vi "INTERFACE.EDIBON.vi"() -> ()   [LabVIEW 2014]
uses:
  Global 5.vi
  <vilib>/measure/madcrms.llb/Basic Averaged DC-RMS for N Chan.vi
  Global 2.vi
  <vilib>/measure/NI_MAPro.lvlib
  <vilib>/Analysis/NI_AALPro.lvlib
panel:
  out "?":dbl format="%#_3f"
  out "?":dbl format="%#_3f"
  out "SRL-1":dbl format="%#_5f"
  out "ST-3":dbl format="%#_4f"
  out "ST-2":dbl format="%#_4f"
  out "V_DC":dbl format="%#_3f"
  out "I_DC":dbl format="%#_3f"
  out "ST-1":dbl format="%#_4f"
  out "I_DC":dbl format="%#_3f"
  out "V_DC":dbl format="%#_3f"
  in  "SOL 2":dbl(slide) min=0.0 max=10.0 step=2.0 scale=0.0..10.0 scale format="%#_1f"
  in  "chave sol2":bool
  in  "chave sol1":bool
  in  "MEAS":bool
  in  "VENTILADORES":bool
  in  "SÉRIE-PARALELO":bool
  out "SRL-1":dbl format="%#_5f"
  out "ST-3":dbl format="%#_4f"
  out "ST-2":dbl format="%#_4f"
  out "ST-1":dbl format="%#_4f"
  in  "PAINEL 2":bool
  in  "PAINEL 1":bool
  in  "SOL 1":dbl(slide) min=0.0 max=10.0 step=2.0 scale=0.0..10.0 scale format="%#_1f"
  in  "stop":bool
  out "Tempo de salvamento (sec)":dbl format="%.1f"
  in  "OK Button":bool
  in  "COMEÇAR":bool
  in  "quit? (T)":bool
  in  "?":bool
  in  "PLOTE NO GRÁFICO:":u16(ring) items=["GRÁFICO A", "GRÁFICO B", "GRÁFICO ÚNICO"]
  in  "I_DC":bool
  in  "ST_2":bool
  in  "ST_1":bool
  in  "V_DC":bool
  in  "ST_3":bool
  in  "SRL_1":bool
  in  "I_DC":bool
  in  "ST_2":bool
  in  "ST_1":bool
  in  "V_DC":bool
  in  "ST_3":bool
  in  "SRL_1":bool
  out "GRÁFICO B":cluster{dbl[], dbl[]}[](graph)
  out "GRÁFICO A":cluster{dbl[], dbl[]}[](graph)
  out "GRÁFICO ÚNICO":cluster{dbl[], dbl[]}[](graph)
  in  "I_DC":bool
  in  "ST_2":bool
  in  "ST_1":bool
  in  "V_DC":bool
  in  "ST_3":bool
  in  "SRL_1":bool
  # "POTENCIA DE SAIDA"
  # "W"
  # "ºC"
  # "ºC"
  # "ºC"
  # "W/m2"
  # "V"
  # "A"
  # "PLOTE O SENSOR:"
  # "ANTES"
  # "DEPOIS"
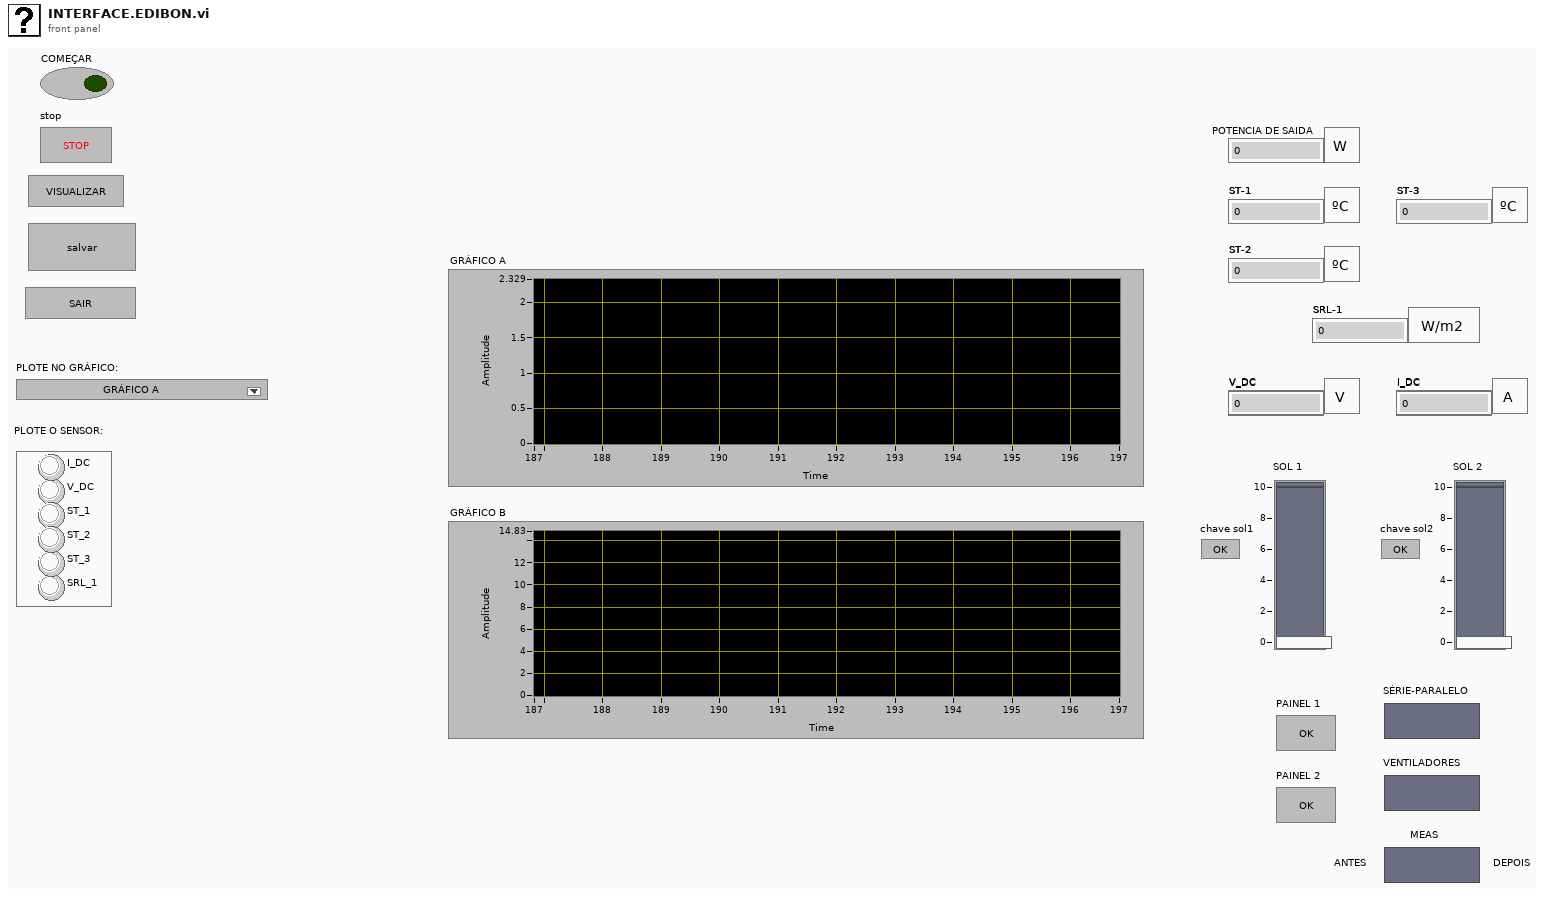
[diagram p1: front panel]
types:
  T1 = enum32{"Invalid", "Standard", "Closed", "Hidden", "Minimized", "Maximized"}
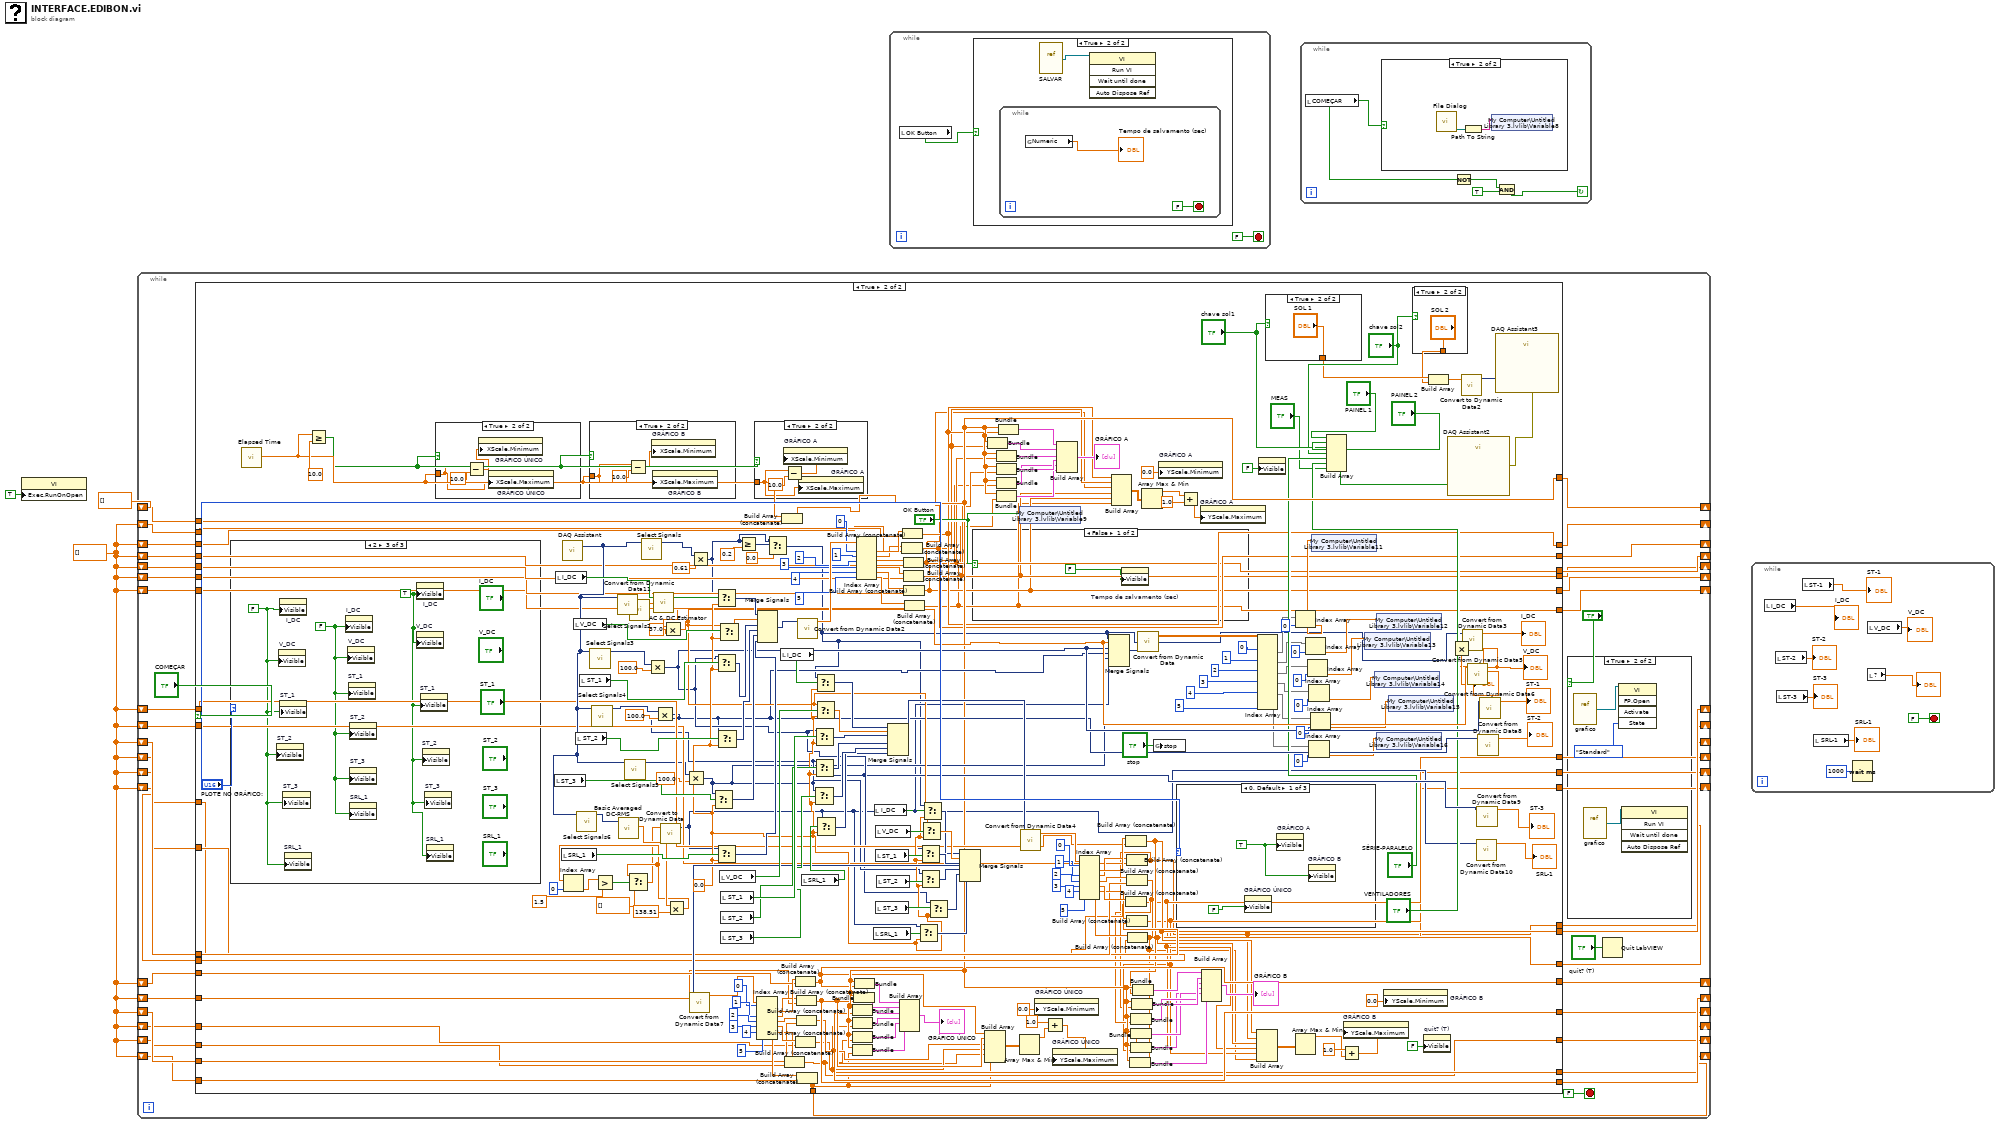
[diagram p0: block diagram]
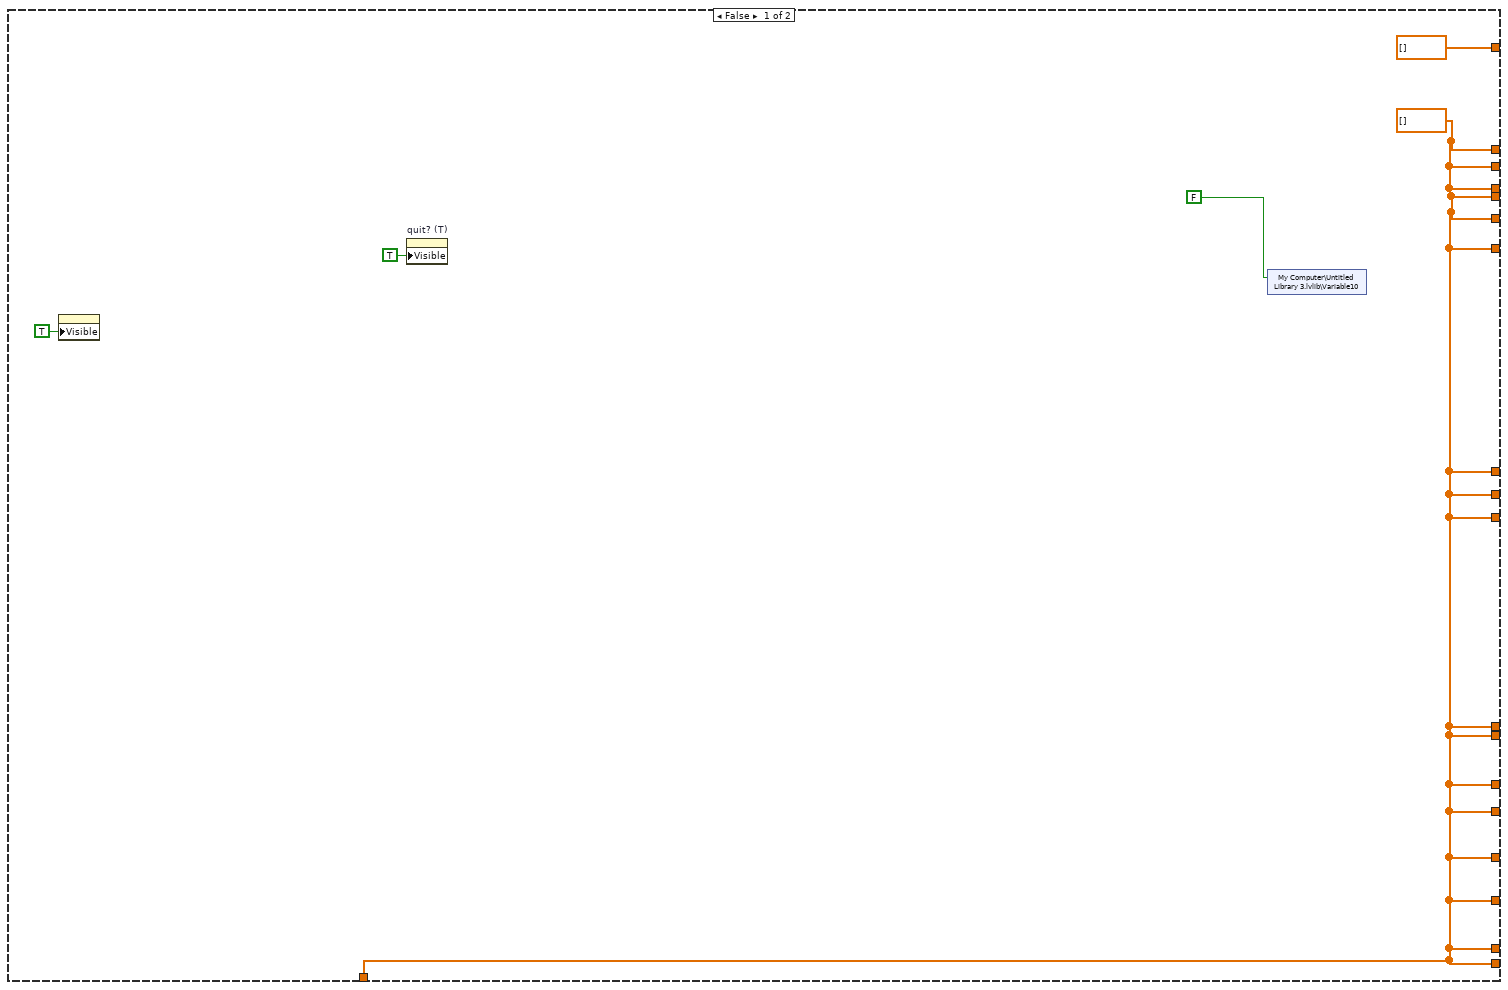
[diagram p5: hidden frame]
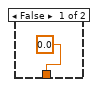
[diagram p6: hidden frame]
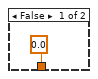
[diagram p7: hidden frame]
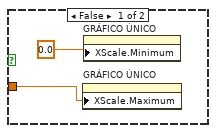
[diagram p8: hidden frame]
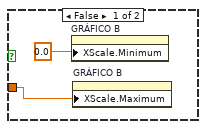
[diagram p9: hidden frame]
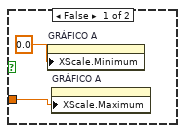
[diagram p10: hidden frame]
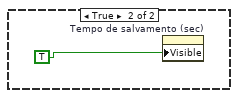
[diagram p11: hidden frame]
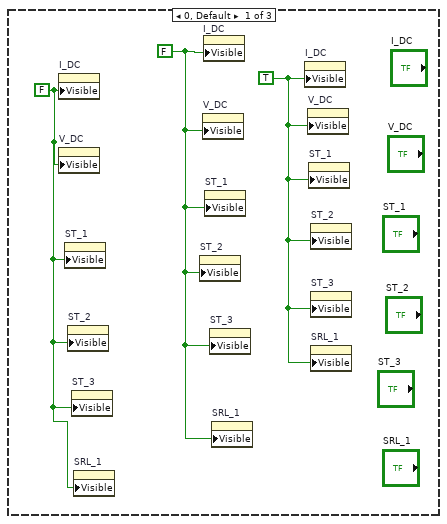
[diagram p12: hidden frame]
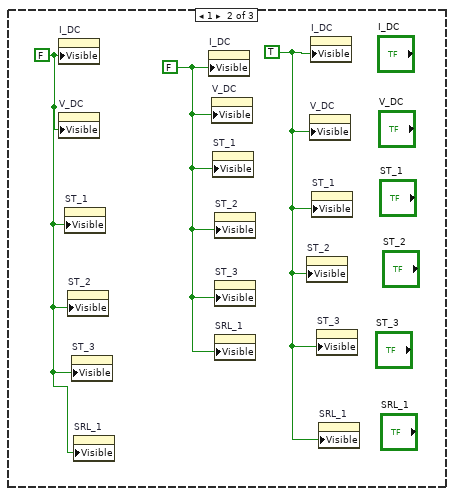
[diagram p13: hidden frame]
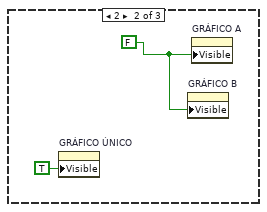
[diagram p14: hidden frame]
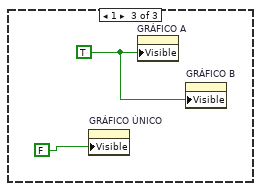
[diagram p15: hidden frame]
diagram:
  w1 = dbl[] []
  n1 = property class="VI"("Exec.RunOnOpen"=TRUE ("Execution:Run When Opened")) -> ()  [unwired: 2 in, 2 out]
  n2 = while {
    shift-right: [w16] -> _
    shift-left: dbl[] [] -> [w17]
    shift-right: [w9] -> _
    shift-left: w1 -> [w15]
    shift-right: [w8] -> _
    shift-left: w1 -> [w14]
    shift-right: [w7] -> _
    shift-left: w1 -> [w13]
    shift-right: [w6] -> _
    shift-left: w1 -> [w12]
    shift-right: [w5] -> _
    shift-left: w1 -> [w11]
    shift-right: [w4] -> _
    shift-left: w1 -> [w10]
    shift-right: [w41] -> _
    shift-left: w1 -> [w40]
    shift-right: [w39] -> _
    shift-left: w1 -> [w38]
    shift-right: [w37] -> _
    shift-left: w1 -> [w33]
    shift-right: [w36] -> _
    shift-left: w1 -> [w32]
    shift-right: [w35] -> _
    shift-left: w1 -> [w31]
    shift-right: [w34] -> _
    shift-left: w1 -> [w30]
    shift-right: [w23] -> _
    shift-left: w1 -> [w29]
    shift-right: [w22] -> _
    shift-left: w1 -> [w28]
    shift-right: [w21] -> _
    shift-left: w1 -> [w27]
    shift-right: [w20] -> _
    shift-left: w1 -> [w26]
    shift-right: [w19] -> _
    shift-left: w1 -> [w25]
    shift-right: [w18] -> _
    shift-left: w1 -> [w24]
    stop <- FALSE stop-if-true
    n3 = case shown="True" "COMEÇAR" {
      tunnel: [dbl[] [] w144] -> w16
      tunnel: [w49 w67] -> w9
      tunnel: [w49 w65] -> w7
      tunnel: [w49 w66] -> w8
      tunnel: [w49 w64] -> w6
      tunnel: [w49 w63] -> w5
      tunnel: [w49 w62] -> w4
      tunnel: [w49 w79] -> w41
      tunnel: w40 -> [_ w217]
      tunnel: [w49 w56] -> w39
      tunnel: w38 -> [_ w216]
      tunnel: [w49 w78] -> w37
      tunnel: [w49 w77] -> w36
      tunnel: [w49 w76] -> w35
      tunnel: [w49 w75] -> w34
      tunnel: w33 -> [_ w215]
      tunnel: w32 -> [_ w214]
      tunnel: w31 -> [_ w213]
      tunnel: w30 -> [_ w212]
      tunnel: w29 -> [_ w191]
      tunnel: w28 -> [_ w190]
      tunnel: w27 -> [_ w189]
      tunnel: w26 -> [_ w188]
      tunnel: w25 -> [_ w187]
      tunnel: w24 -> [_ w186]
      tunnel: [w49 w86] -> w23
      tunnel: [w49 w85] -> w22
      tunnel: [w49 w84] -> w21
      tunnel: [w49 w83] -> w20
      tunnel: [w49 w82] -> w19
      tunnel: [w49 w81] -> w18
      tunnel: w17 -> [_ w145]
      tunnel: w15 -> [_ w143]
      tunnel: w14 -> [_ w142]
      tunnel: w13 -> [_ w141]
      tunnel: w12 -> [_ w140]
      tunnel: w11 -> [_ w139]
      tunnel: w10 -> [_ w138]
      frame False {
        w49 = dbl[] []
        n4 = property class="Bool"("Visible"=TRUE) -> ()  [unwired: 2 in, 2 out]
        n5 = property on="quit? (T)" class="Bool (strict)"("Visible"=TRUE) -> ()  [unwired: 2 in, 2 out]
        n6 = shared-variable "My Computer\\Untitled Library 3.lvlib\\Variable10"(FALSE ("Variable5")) -> ()  [unwired: 1 in, 1 out]
      }
      frame True {
        w242 = 0.0
        n7 = case shown="2" "PLOTE NO GRÁFICO:" {
          frame 0, Default {
            w315 = FALSE ("Visible")
            w316 = TRUE ("Visible")
            w317 = FALSE ("Visible")
            n8 = property on="I_DC" class="Bool (strict)"("Visible"=w315) -> ()  [unwired: 2 in, 2 out]
            n9 = property on="V_DC" class="Bool (strict)"("Visible"=w315) -> ()  [unwired: 2 in, 2 out]
            n10 = property on="ST_1" class="Bool (strict)"("Visible"=w315) -> ()  [unwired: 2 in, 2 out]
            n11 = property on="ST_2" class="Bool (strict)"("Visible"=w315) -> ()  [unwired: 2 in, 2 out]
            n12 = property on="ST_3" class="Bool (strict)"("Visible"=w315) -> ()  [unwired: 2 in, 2 out]
            n13 = property on="SRL_1" class="Bool (strict)"("Visible"=w315) -> ()  [unwired: 2 in, 2 out]
            n14 = property on="ST_2" class="Bool (strict)"("Visible"=w317) -> ()  [unwired: 2 in, 2 out]
            n15 = property on="V_DC" class="Bool (strict)"("Visible"=w317) -> ()  [unwired: 2 in, 2 out]
            n16 = property on="I_DC" class="Bool (strict)"("Visible"=w317) -> ()  [unwired: 2 in, 2 out]
            n17 = property on="ST_1" class="Bool (strict)"("Visible"=w317) -> ()  [unwired: 2 in, 2 out]
            n18 = property on="ST_3" class="Bool (strict)"("Visible"=w317) -> ()  [unwired: 2 in, 2 out]
            n19 = property on="SRL_1" class="Bool (strict)"("Visible"=w317) -> ()  [unwired: 2 in, 2 out]
            n20 = property on="I_DC" class="Bool (strict)"("Visible"=w316) -> ()  [unwired: 2 in, 2 out]
            n21 = property on="V_DC" class="Bool (strict)"("Visible"=w316) -> ()  [unwired: 2 in, 2 out]
            n22 = property on="ST_1" class="Bool (strict)"("Visible"=w316) -> ()  [unwired: 2 in, 2 out]
            n23 = property on="ST_2" class="Bool (strict)"("Visible"=w316) -> ()  [unwired: 2 in, 2 out]
            n24 = property on="ST_3" class="Bool (strict)"("Visible"=w316) -> ()  [unwired: 2 in, 2 out]
            n25 = property on="SRL_1" class="Bool (strict)"("Visible"=w316) -> ()  [unwired: 2 in, 2 out]
          }
          frame 1 {
            w318 = FALSE ("Visible")
            w319 = TRUE ("Visible")
            w320 = FALSE ("Visible")
            n26 = property on="I_DC" class="Bool (strict)"("Visible"=w318) -> ()  [unwired: 2 in, 2 out]
            n27 = property on="V_DC" class="Bool (strict)"("Visible"=w318) -> ()  [unwired: 2 in, 2 out]
            n28 = property on="ST_1" class="Bool (strict)"("Visible"=w318) -> ()  [unwired: 2 in, 2 out]
            n29 = property on="ST_2" class="Bool (strict)"("Visible"=w318) -> ()  [unwired: 2 in, 2 out]
            n30 = property on="ST_3" class="Bool (strict)"("Visible"=w318) -> ()  [unwired: 2 in, 2 out]
            n31 = property on="SRL_1" class="Bool (strict)"("Visible"=w318) -> ()  [unwired: 2 in, 2 out]
            n32 = property on="I_DC" class="Bool (strict)"("Visible"=w320) -> ()  [unwired: 2 in, 2 out]
            n33 = property on="V_DC" class="Bool (strict)"("Visible"=w320) -> ()  [unwired: 2 in, 2 out]
            n34 = property on="ST_1" class="Bool (strict)"("Visible"=w320) -> ()  [unwired: 2 in, 2 out]
            n35 = property on="ST_2" class="Bool (strict)"("Visible"=w320) -> ()  [unwired: 2 in, 2 out]
            n36 = property on="ST_3" class="Bool (strict)"("Visible"=w320) -> ()  [unwired: 2 in, 2 out]
            n37 = property on="SRL_1" class="Bool (strict)"("Visible"=w320) -> ()  [unwired: 2 in, 2 out]
            n38 = property on="ST_2" class="Bool (strict)"("Visible"=w319) -> ()  [unwired: 2 in, 2 out]
            n39 = property on="V_DC" class="Bool (strict)"("Visible"=w319) -> ()  [unwired: 2 in, 2 out]
            n40 = property on="I_DC" class="Bool (strict)"("Visible"=w319) -> ()  [unwired: 2 in, 2 out]
            n41 = property on="ST_1" class="Bool (strict)"("Visible"=w319) -> ()  [unwired: 2 in, 2 out]
            n42 = property on="ST_3" class="Bool (strict)"("Visible"=w319) -> ()  [unwired: 2 in, 2 out]
            n43 = property on="SRL_1" class="Bool (strict)"("Visible"=w319) -> ()  [unwired: 2 in, 2 out]
          }
          frame 2 {
            w321 = FALSE ("Visible")
            w322 = FALSE ("Visible")
            w323 = TRUE ("Visible")
            n44 = property on="ST_2" class="Bool (strict)"("Visible"=w322) -> ()  [unwired: 2 in, 2 out]
            n45 = property on="V_DC" class="Bool (strict)"("Visible"=w322) -> ()  [unwired: 2 in, 2 out]
            n46 = property on="I_DC" class="Bool (strict)"("Visible"=w322) -> ()  [unwired: 2 in, 2 out]
            n47 = property on="ST_1" class="Bool (strict)"("Visible"=w322) -> ()  [unwired: 2 in, 2 out]
            n48 = property on="ST_3" class="Bool (strict)"("Visible"=w322) -> ()  [unwired: 2 in, 2 out]
            n49 = property on="SRL_1" class="Bool (strict)"("Visible"=w322) -> ()  [unwired: 2 in, 2 out]
            n50 = property on="I_DC" class="Bool (strict)"("Visible"=w321) -> ()  [unwired: 2 in, 2 out]
            n51 = property on="V_DC" class="Bool (strict)"("Visible"=w321) -> ()  [unwired: 2 in, 2 out]
            n52 = property on="ST_1" class="Bool (strict)"("Visible"=w321) -> ()  [unwired: 2 in, 2 out]
            n53 = property on="ST_2" class="Bool (strict)"("Visible"=w321) -> ()  [unwired: 2 in, 2 out]
            n54 = property on="ST_3" class="Bool (strict)"("Visible"=w321) -> ()  [unwired: 2 in, 2 out]
            n55 = property on="SRL_1" class="Bool (strict)"("Visible"=w321) -> ()  [unwired: 2 in, 2 out]
            n56 = property on="I_DC" class="Bool (strict)"("Visible"=w323) -> ()  [unwired: 2 in, 2 out]
            n57 = property on="V_DC" class="Bool (strict)"("Visible"=w323) -> ()  [unwired: 2 in, 2 out]
            n58 = property on="ST_1" class="Bool (strict)"("Visible"=w323) -> ()  [unwired: 2 in, 2 out]
            n59 = property on="ST_2" class="Bool (strict)"("Visible"=w323) -> ()  [unwired: 2 in, 2 out]
            n60 = property on="ST_3" class="Bool (strict)"("Visible"=w323) -> ()  [unwired: 2 in, 2 out]
            n61 = property on="SRL_1" class="Bool (strict)"("Visible"=w323) -> ()  [unwired: 2 in, 2 out]
          }
        }
        n62 = call "Elapsed Time"() -> ("Elapsed Time (s)"=w232:dbl)  [unwired: 12 in, 7 out]
        n63 = Greater Or Equal?(x=w232, y=10.0) -> (x >= y?=w231:bool)
        n64 = case shown="True" w231 {
          tunnel: w232 -> [w298 w300]
          frame False {
            n65 = property on="GRÁFICO ÚNICO" class="XYGraph (strict)"("XScale.Maximum"=w298) -> ()  [unwired: 2 in, 2 out]
            n66 = property on="GRÁFICO ÚNICO" class="XYGraph (strict)"("XScale.Minimum"=0.0 ("X Scale.Range:Minimum")) -> ()  [unwired: 2 in, 2 out]
          }
          frame True {
            n67 = Subtract(x=w300, y=10.0) -> (x-y=w301:dbl)
            n68 = property on="GRÁFICO ÚNICO" class="XYGraph (strict)"("XScale.Minimum"=w301) -> ()  [unwired: 2 in, 2 out]
            n69 = property on="GRÁFICO ÚNICO" class="XYGraph (strict)"("XScale.Maximum"=w300) -> ()  [unwired: 2 in, 2 out]
          }
        }
        n70 = local read "ST_3"() -> (w280:bool)
        n71 = local read "I_DC"() -> (w283:bool)
        n72 = local read "SRL_1"() -> (w281:bool)
        n73 = call "DAQ Assistant"() -> ("data"=w248:dynamicdata)  [unwired: 16 in, 3 out]
        n74 = local read "V_DC"() -> (w282:bool)
        n75 = local read "ST_2"() -> (w279:bool)
        n76 = call "Select Signals6"("Signals"=w248) -> ("Signal Out"=w110:dynamicdata)  [unwired: 9 in, 1 out]
        n77 = local read "ST_1"() -> (w278:bool)
        n78 = case shown="True" w231 {
          tunnel: w232 -> [w303 w306]
          frame False {
            n79 = property on="GRÁFICO B" class="XYGraph (strict)"("XScale.Minimum"=0.0 ("X Scale.Range:Minimum")) -> ()  [unwired: 2 in, 2 out]
            n80 = property on="GRÁFICO B" class="XYGraph (strict)"("XScale.Maximum"=w303) -> ()  [unwired: 2 in, 2 out]
          }
          frame True {
            n81 = Subtract(x=w306, y=10.0) -> (x-y=w305:dbl)
            n82 = property on="GRÁFICO B" class="XYGraph (strict)"("XScale.Minimum"=w305) -> ()  [unwired: 2 in, 2 out]
            n83 = property on="GRÁFICO B" class="XYGraph (strict)"("XScale.Maximum"=w306) -> ()  [unwired: 2 in, 2 out]
          }
        }
        n84 = call "Select Signals3"("Signals"=w248) -> ("Signal Out"=w164:dynamicdata)  [unwired: 9 in, 1 out]
        n85 = call "Select Signals4"("Signals"=w248) -> ("Signal Out"=w162:dynamicdata)  [unwired: 9 in, 1 out]
        n86 = call "Select Signals2"("Signals"=w248) -> ("Signal Out"=w105:dynamicdata)  [unwired: 9 in, 1 out]
        n87 = call-poly <vilib>:"Basic Averaged DC-RMS.vi"("signals in"=w110) -> ("RMS values"=w106:dbl[])  [unwired: 7 in, 3 out]
        n88 = call "Select Signals5"("Signals"=w248) -> ("Signal Out"=w160:dynamicdata)  [unwired: 9 in, 1 out]
        n89 = call "Convert from Dynamic Data11"("Dynamic Data Type"=w105) -> ("Array"=w104:dbl[])  [unwired: 3 in]
        n90 = call "Select Signals"("Signals"=w248) -> ("Signal Out"=w166:dynamicdata)  [unwired: 9 in, 1 out]
        n91 = Multiply(x=w164, y=100.0) -> (x*y=w158:dynamicdata)
        n92 = call <vilib>:"AC & DC Estimator.vi"("Signal (V)"=w104) -> ("DC estimate (V)"=w103:dbl)  [unwired: 1 out]
        n93 = Multiply(x=w162, y=100.0) -> (x*y=w156:dynamicdata)
        n94 = Multiply(x=w103, y=37.0) -> (x*y=w159:dbl)
        n95 = Multiply(x=w106, y=138.51) -> (x*y=w97:dbl[])
        n96 = Index Array(array=w97, index=0) -> (element=w100:dbl)
        n97 = Greater?(x=w100, y=1.5) -> (0:w98:bool)
        n98 = Select(t=w97, s=w98, f=dbl[] []) -> (s? t:f=w96:dbl[])
        n99 = call "Convert to Dynamic Data"("Array"=w96) -> ("Dynamic Data Type"=w109:dynamicdata)  [unwired: 3 in]
        n100 = Multiply(x=w160, y=100.0) -> (x*y=w154:dynamicdata)
        n101 = Multiply(x=w166, y=0.61) -> (x*y=w92:dynamicdata)
        n102 = Select(t=w154, s=w280, f=w242) -> (s? t:f=w290:dynamicdata)
        n103 = Select(t=w92, s=w283, f=w242) -> (s? t:f=w247:dynamicdata)
        n104 = Select(t=w158, s=w278, f=w242) -> (s? t:f=w292:dynamicdata)
        n105 = Select(t=w109, s=w281, f=w242) -> (s? t:f=w289:dynamicdata)
        n106 = Select(t=w156, s=w279, f=w242) -> (s? t:f=w291:dynamicdata)
        n107 = Select(t=w159, s=w282, f=w242) -> (s? t:f=w293:dbl)
        n108 = local read "V_DC"() -> (w276:bool)
        n109 = local read "ST_1"() -> (w275:bool)
        n110 = local read "ST_2"() -> (w274:bool)
        n111 = local read "ST_3"() -> (w273:bool)
        n112 = Greater Or Equal?(x=w92, y=0.2) -> (x >= y?=w93:dynamicdata)
        n113 = case shown="True" w231 {
          tunnel: w232 -> [w309 w310]
          frame False {
            n114 = property on="GRÁFICO A" class="XYGraph (strict)"("XScale.Minimum"=0.0 ("X Scale.Range:Minimum")) -> ()  [unwired: 2 in, 2 out]
            n115 = property on="GRÁFICO A" class="XYGraph (strict)"("XScale.Maximum"=w309) -> ()  [unwired: 2 in, 2 out]
          }
          frame True {
            n116 = Subtract(x=w310, y=10.0) -> (x-y=w311:dbl)
            n117 = property on="GRÁFICO A" class="XYGraph (strict)"("XScale.Minimum"=w311) -> ()  [unwired: 2 in, 2 out]
            n118 = property on="GRÁFICO A" class="XYGraph (strict)"("XScale.Maximum"=w310) -> ()  [unwired: 2 in, 2 out]
          }
        }
        n119 = Merge Signals(w247, w293, w292, w291, w290, w289) -> (w236:dynamicdata)
        n120 = Select(t=w92, s=w93, f=0.0) -> (s? t:f=w90:dynamicdata)
        n121 = local read "I_DC"() -> (w277:bool)
        n122 = Build Array (concatenate)(w232, w145) -> (w144:dbl[])
        n123 = call "Convert from Dynamic Data2"("Dynamic Data Type"=w236) -> ("Array"=w239:dbl[])  [unwired: 3 in]
        n124 = local read "SRL_1"() -> (w272:bool)
        n125 = Select(t=w154, s=w273, f=w242) -> (s? t:f=w285:dynamicdata)
        n126 = Select(t=w158, s=w275, f=w242) -> (s? t:f=w287:dynamicdata)
        n127 = Select(t=w156, s=w274, f=w242) -> (s? t:f=w286:dynamicdata)
        n128 = Select(t=w90, s=w277, f=w242) -> (s? t:f=w244:dynamicdata)
        n129 = Select(t=w159, s=w276, f=w242) -> (s? t:f=w288:dbl)
        n130 = Select(t=w109, s=w272, f=w242) -> (s? t:f=w284:dynamicdata)
        n131 = Index Array(array=w239, index #1=0 ("index"), index #2=1 ("index"), index #3=2 ("index"), index #4=3 ("index"), index #5=4 ("index"), index #6=5 ("index")) -> (element #1=w151:dbl, element #2=w150:dbl, element #3=w149:dbl, element #4=w148:dbl, element #5=w147:dbl, element #6=w146:dbl)
        n132 = local read "SRL_1"() -> (w266:bool)
        n133 = local read "I_DC"() -> (w271:bool)
        n134 = local read "V_DC"() -> (w270:bool)
        n135 = local read "ST_1"() -> (w269:bool)
        n136 = local read "ST_3"() -> (w267:bool)
        n137 = local read "ST_2"() -> (w268:bool)
        n138 = Merge Signals(w244, w288, w287, w286, w285, w284) -> (w246:dynamicdata)
        n139 = Build Array (concatenate)(w150, w142) -> (w66:dbl[])
        n140 = Build Array (concatenate)(w151, w143) -> (w67:dbl[])
        n141 = Build Array (concatenate)(w149, w141) -> (w65:dbl[])
        n142 = Build Array (concatenate)(w148, w140) -> (w64:dbl[])
        n143 = Build Array (concatenate)(w147, w139) -> (w63:dbl[])
        n144 = Build Array (concatenate)(w146, w138) -> (w62:dbl[])
        n145 = Select(t=w109, s=w266, f=w242) -> (s? t:f=w261:dynamicdata)
        n146 = Select(t=w158, s=w269, f=w242) -> (s? t:f=w264:dynamicdata)
        n147 = Select(t=w156, s=w268, f=w242) -> (s? t:f=w263:dynamicdata)
        n148 = Select(t=w159, s=w270, f=w242) -> (s? t:f=w265:dbl)
        n149 = Select(t=w90, s=w271, f=w242) -> (s? t:f=w243:dynamicdata)
        n150 = Select(t=w154, s=w267, f=w242) -> (s? t:f=w262:dynamicdata)
        n151 = Merge Signals(w243, w265, w264, w263, w262, w261) -> (w245:dynamicdata)
        n152 = call "Convert from Dynamic Data7"("Dynamic Data Type"=w245) -> ("Array"=w198:dbl[])  [unwired: 3 in]
        n153 = Index Array(array=w198, index #1=0 ("index"), index #2=1 ("index"), index #3=2 ("index"), index #4=3 ("index"), index #5=4 ("index"), index #6=5 ("index")) -> (element #1=w197:dbl, element #2=w196:dbl, element #3=w195:dbl, element #4=w194:dbl, element #5=w193:dbl, element #6=w192:dbl)
        n154 = Build Array (concatenate)(w193, w187) -> (w82:dbl[])
        n155 = Build Array (concatenate)(w197, w191) -> (w86:dbl[])
        n156 = Build Array (concatenate)(w194, w188) -> (w83:dbl[])
        n157 = Build Array (concatenate)(w196, w190) -> (w85:dbl[])
        n158 = Build Array (concatenate)(w195, w189) -> (w84:dbl[])
        n159 = Build Array (concatenate)(w192, w186) -> (w81:dbl[])
        n160 = Bundle(w144, w84) -> (w183:cluster{dbl[], dbl[]})  [unwired: 1 in]
        n161 = Bundle(w144, w83) -> (w182:cluster{dbl[], dbl[]})  [unwired: 1 in]
        n162 = Bundle(w144, w82) -> (w181:cluster{dbl[], dbl[]})  [unwired: 1 in]
        n163 = Bundle(w144, w81) -> (w180:cluster{dbl[], dbl[]})  [unwired: 1 in]
        n164 = Bundle(w144, w85) -> (w184:cluster{dbl[], dbl[]})  [unwired: 1 in]
        n165 = Bundle(w144, w86) -> (w185:cluster{dbl[], dbl[]})  [unwired: 1 in]
        n166 = Build Array(w185, w184, w183, w182, w181, w180) -> (→"GRÁFICO ÚNICO":cluster{dbl[], dbl[]}[])
        n167 = case shown="False" "OK Button" {
          frame False {
            n168 = property on="Tempo de salvamento (sec)" class="DigNum (strict)"("Visible"=FALSE) -> ()  [unwired: 2 in, 2 out]
          }
          frame True {
            n169 = property on="Tempo de salvamento (sec)" class="DigNum (strict)"("Visible"=TRUE) -> ()  [unwired: 2 in, 2 out]
          }
        }
        n170 = Build Array(w86, w85, w84, w83, w82, w81) -> (w80:dbl[][])
        n171 = Bundle(w144, w66) -> (w136:cluster{dbl[], dbl[]})  [unwired: 1 in]
        n172 = Bundle(w144, w65) -> (w135:cluster{dbl[], dbl[]})  [unwired: 1 in]
        n173 = Bundle(w144, w64) -> (w134:cluster{dbl[], dbl[]})  [unwired: 1 in]
        n174 = Bundle(w144, w63) -> (w133:cluster{dbl[], dbl[]})  [unwired: 1 in]
        n175 = Bundle(w144, w62) -> (w132:cluster{dbl[], dbl[]})  [unwired: 1 in]
        n176 = Bundle(w144, w67) -> (w137:cluster{dbl[], dbl[]})  [unwired: 1 in]
        n177 = shared-variable "My Computer\\Untitled Library 3.lvlib\\Variable9"("OK Button") -> ()  [unwired: 1 in, 1 out]
        n178 = Array Max & Min(array=w80) -> (max value=w73:dbl)  [unwired: 3 out]
        n179 = call "Convert from Dynamic Data4"("Dynamic Data Type"=w246) -> ("Array"=w224:dbl[])  [unwired: 3 in]
        n180 = property on="GRÁFICO ÚNICO" class="XYGraph (strict)"("YScale.Minimum"=0.0 ("Y Scale.Range:Minimum")) -> ()  [unwired: 2 in, 2 out]
        n181 = Add(x=1.0, y=w73) -> (x+y=w71:dbl)
        n182 = property on="GRÁFICO ÚNICO" class="XYGraph (strict)"("YScale.Maximum"=w71) -> ()  [unwired: 2 in, 2 out]
        n183 = Build Array(w137, w136, w135, w134, w133, w132) -> (→"GRÁFICO A":cluster{dbl[], dbl[]}[])
        n184 = Index Array(array=w224, index #1=0 ("index"), index #2=1 ("index"), index #3=2 ("index"), index #4=3 ("index"), index #5=4 ("index"), index #6=5 ("index")) -> (element #1=w223:dbl, element #2=w222:dbl, element #3=w221:dbl, element #4=w220:dbl, element #5=w219:dbl, element #6=w218:dbl)
        n185 = Merge Signals(w90, w159, w158, w156, w154, w109) -> (w258:dynamicdata)
        n186 = Build Array(w67, w66, w65, w64, w63, w62) -> (w61:dbl[][])
        n187 = Build Array (concatenate)(w223, w217) -> (w79:dbl[])
        n188 = Build Array (concatenate)(w220, w214) -> (w77:dbl[])
        n189 = Build Array (concatenate)(w222, w216) -> (w56:dbl[])
        n190 = Build Array (concatenate)(w221, w215) -> (w78:dbl[])
        n191 = Build Array (concatenate)(w219, w213) -> (w76:dbl[])
        n192 = Build Array (concatenate)(w218, w212) -> (w75:dbl[])
        n193 = Bundle(w144, w75) -> (w206:cluster{dbl[], dbl[]})  [unwired: 1 in]
        n194 = Bundle(w144, w78) -> (w209:cluster{dbl[], dbl[]})  [unwired: 1 in]
        n195 = Bundle(w144, w77) -> (w208:cluster{dbl[], dbl[]})  [unwired: 1 in]
        n196 = Bundle(w144, w76) -> (w207:cluster{dbl[], dbl[]})  [unwired: 1 in]
        n197 = Bundle(w144, w56) -> (w210:cluster{dbl[], dbl[]})  [unwired: 1 in]
        n198 = Bundle(w144, w79) -> (w211:cluster{dbl[], dbl[]})  [unwired: 1 in]
        n199 = call "Convert from Dynamic Data"("Dynamic Data Type"=w258) -> ("Array"=w257:dbl[][])  [unwired: 3 in]
        n200 = Array Max & Min(array=w61) -> (max value=w59:dbl)  [unwired: 3 out]
        n201 = global write "Global 5.vi" "stop"("stop") -> ()
        n202 = property on="GRÁFICO A" class="XYGraph (strict)"("YScale.Minimum"=0.0 ("Y Scale.Range:Minimum")) -> ()  [unwired: 2 in, 2 out]
        n203 = case shown="0, Default" "PLOTE NO GRÁFICO:" {
          frame 0, Default {
            w325 = TRUE ("Visible")
            n204 = property on="GRÁFICO ÚNICO" class="XYGraph (strict)"("Visible"=FALSE) -> ()  [unwired: 2 in, 2 out]
            n205 = property on="GRÁFICO A" class="XYGraph (strict)"("Visible"=w325) -> ()  [unwired: 2 in, 2 out]
            n206 = property on="GRÁFICO B" class="XYGraph (strict)"("Visible"=w325) -> ()  [unwired: 2 in, 2 out]
          }
          frame 2 {
            w326 = FALSE ("Visible")
            n207 = property on="GRÁFICO ÚNICO" class="XYGraph (strict)"("Visible"=TRUE) -> ()  [unwired: 2 in, 2 out]
            n208 = property on="GRÁFICO B" class="XYGraph (strict)"("Visible"=w326) -> ()  [unwired: 2 in, 2 out]
            n209 = property on="GRÁFICO A" class="XYGraph (strict)"("Visible"=w326) -> ()  [unwired: 2 in, 2 out]
          }
          frame 1 {
            w329 = TRUE ("Visible")
            n210 = property on="GRÁFICO ÚNICO" class="XYGraph (strict)"("Visible"=FALSE) -> ()  [unwired: 2 in, 2 out]
            n211 = property on="GRÁFICO A" class="XYGraph (strict)"("Visible"=w329) -> ()  [unwired: 2 in, 2 out]
            n212 = property on="GRÁFICO B" class="XYGraph (strict)"("Visible"=w329) -> ()  [unwired: 2 in, 2 out]
          }
        }
        n213 = Add(x=w59, y=1.0) -> (x+y=w58:dbl)
        n214 = property on="GRÁFICO A" class="XYGraph (strict)"("YScale.Maximum"=w58) -> ()  [unwired: 2 in, 2 out]
        n215 = Build Array(w211, w210, w209, w208, w207, w206) -> (→"GRÁFICO B":cluster{dbl[], dbl[]}[])
        n216 = Build Array(w79, w56, w78, w77, w76, w75) -> (w74:dbl[][])
        n217 = Index Array(array=w257, index (row) #1=0 ("index"), index (row) #2=1 ("index"), index (row) #3=2 ("index"), index (row) #4=3 ("index"), index (row) #5=4 ("index"), index (row) #6=5 ("index (row)")) -> (element #1=w129:dbl[], element #2=w124:dbl[], element #3=w123:dbl[], element #4=w118:dbl[], element #5=w117:dbl[], element #6=w113:dbl[])  [unwired: 6 in]
        n218 = property class="Bool"("Visible"=FALSE) -> ()  [unwired: 2 in, 2 out]
        n219 = case shown="True" "chave sol1" {
          tunnel: [0.0 ("SOL 1") "SOL 1"] -> w172
          frame False {
          }
          frame True {
          }
        }
        n220 = Index Array(array=w129, index=0) -> (element=w127:dbl)
        n221 = Array Max & Min(array=w74) -> (max value=w69:dbl)  [unwired: 3 out]
        n222 = Index Array(array=w124, index=0) -> (element=w122:dbl)
        n223 = Index Array(array=w123, index=0) -> (element=w121:dbl)
        n224 = Index Array(array=w118, index=0) -> (element=w116:dbl)
        n225 = Index Array(array=w113, index=0) -> (element=w112:dbl)
        n226 = Index Array(array=w117, index=0) -> (element=w115:dbl)
        n227 = shared-variable "My Computer\\Untitled Library 3.lvlib\\Variable11"(w127) -> ()  [unwired: 1 in, 1 out]
        n228 = Build Array("PAINEL 1", "PAINEL 2", "chave sol1", "chave sol2", "SÉRIE-PARALELO", "VENTILADORES", "MEAS") -> (w177:bool[])
        n229 = Add(x=1.0, y=w69) -> (x+y=w68:dbl)
        n230 = property on="GRÁFICO B" class="XYGraph (strict)"("YScale.Maximum"=w68) -> ()  [unwired: 2 in, 2 out]
        n231 = shared-variable "My Computer\\Untitled Library 3.lvlib\\Variable13"(w121) -> ()  [unwired: 1 in, 1 out]
        n232 = shared-variable "My Computer\\Untitled Library 3.lvlib\\Variable14"(w116) -> ()  [unwired: 1 in, 1 out]
        n233 = shared-variable "My Computer\\Untitled Library 3.lvlib\\Variable12"(w122) -> ()  [unwired: 1 in, 1 out]
        n234 = shared-variable "My Computer\\Untitled Library 3.lvlib\\Variable16"(w112) -> ()  [unwired: 1 in, 1 out]
        n235 = property on="GRÁFICO B" class="XYGraph (strict)"("YScale.Minimum"=0.0 ("Y Scale.Range:Minimum")) -> ()  [unwired: 2 in, 2 out]
        n236 = shared-variable "My Computer\\Untitled Library 3.lvlib\\Variable15"(w115) -> ()  [unwired: 1 in, 1 out]
        n237 = case shown="True" "chave sol2" {
          tunnel: [0.0 ("SOL 1") "SOL 2"] -> w171
          frame False {
          }
          frame True {
          }
        }
        n238 = property on="quit? (T)" class="Bool (strict)"("Visible"=FALSE) -> ()  [unwired: 2 in, 2 out]
        n239 = Build Array(w172, w171) -> (w170:dbl[])
        n240 = call "DAQ Assistant2"("data"=w177) -> ("error out"=w174:errorcluster)  [unwired: 17 in, 1 out]
        n241 = call "Convert to Dynamic Data2"("Array"=w170) -> ("Dynamic Data Type"=w169:dynamicdata)  [unwired: 3 in]
        n242 = call "Convert from Dynamic Data3"("Dynamic Data Type"=w90) -> ("Scalar"=w57:dbl)  [unwired: 3 in]
        "I_DC" <- w57
        n243 = call "Convert from Dynamic Data5"("Dynamic Data Type"=w159) -> ("Scalar"=w54:dbl)  [unwired: 3 in]
        "V_DC" <- w54
        n244 = Multiply(x=w57, y=w54) -> (x*y=→"?":dbl)
        n245 = call "Convert from Dynamic Data10"("Dynamic Data Type"=w109) -> ("Scalar"=→"SRL-1":dbl)  [unwired: 3 in]
        n246 = call "Convert from Dynamic Data9"("Dynamic Data Type"=w154) -> ("Scalar"=→"ST-3":dbl)  [unwired: 3 in]
        n247 = call "Convert from Dynamic Data8"("Dynamic Data Type"=w156) -> ("Scalar"=→"ST-2":dbl)  [unwired: 3 in]
        n248 = call "Convert from Dynamic Data6"("Dynamic Data Type"=w158) -> ("Scalar"=→"ST-1":dbl)  [unwired: 3 in]
        n249 = call "DAQ Assistant3"("data"=w169, "error in"=w174) -> ()  [unwired: 16 in, 2 out]
      }
    }
    n250 = case shown="True" "?" {
      frame False {
      }
      frame True {
        n251 = vi-ref "grafico.vi"() -> (w47:refnum<vi>)
        n252 = vi-ref "grafico.vi"() -> (w46:refnum<vi>)
        n253 = invoke class="VI" method="FP.Open"(reference=w47, "State"=T1."Standard") -> ()  [unwired: 3 in, 5 out]
        n254 = invoke class="VI" method="Run VI"(reference=w46) -> ()  [unwired: 4 in, 5 out]
      }
    }
    n255 = Quit LabVIEW(quit? (T)="quit? (T)") -> ()
  }
  n256 = while {
    stop <- FALSE stop-if-true
    n257 = local read "OK Button"() -> (w331:bool)
    n258 = case shown="True" w331 {
      frame False {
      }
      frame True {
        n259 = while {
          stop <- FALSE stop-if-true
          n260 = global read "Global 2.vi" "Numeric"() -> (→"Tempo de salvamento (sec)":dbl)
        }
        n261 = vi-ref "SALVAR.vi"() -> (w332:refnum<vi>)
        n262 = invoke class="VI" method="Run VI"(reference=w332) -> ()  [unwired: 4 in, 5 out]
      }
    }
  }
  n263 = while {
    stop <- w338 continue-if-true
    n264 = local read "COMEÇAR"() -> (w336:bool)
    n265 = case shown="True" w336 {
      frame False {
      }
      frame True {
        n266 = call "File Dialog"() -> ("selected path"=w340:path)  [unwired: 12 in, 3 out]
        n267 = Path To String(path=w340) -> (string=w339:string)
        n268 = shared-variable "My Computer\\Untitled Library 3.lvlib\\Variable8"(w339) -> ()  [unwired: 1 in, 1 out]
      }
    }
    n269 = Not(x=w336) -> (.not. x?=w335:bool)
    n270 = And(x=w335, y=TRUE) -> (x .and. y?=w338:bool)
  }
  n271 = while {
    stop <- FALSE stop-if-true
    n272 = local read "I_DC"() -> (→"I_DC":dbl)
    n273 = local read "ST-2"() -> (→"ST-2":dbl)
    n274 = local read "ST-3"() -> (→"ST-3":dbl)
    n275 = local read "ST-1"() -> (→"ST-1":dbl)
    n276 = local read "SRL-1"() -> (→"SRL-1":dbl)
    n277 = Wait (ms)(milliseconds to wait=u32 1000) -> ()  [unwired: 1 out]
    n278 = local read "V_DC"() -> (→"V_DC":dbl)
    n279 = local read item#49() -> (→"?":dbl)
  }
